vi "chart.vi"() -> ()   [LabVIEW 8.6]
uses:
  Controls/lxw_chart_type.ctl
  Controls/lxw_boolean.ctl
  Controls/lxw_defined_colors.ctl
panel:
  out "error out":errorcluster
  out "function return 2":string
  # "chart.xlsx"
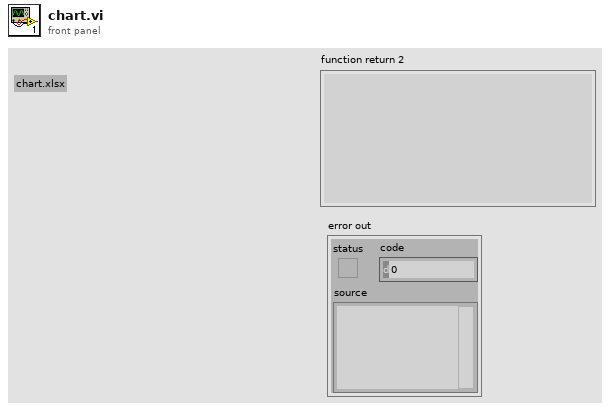
[diagram p1: front panel]
types:
  T1 = typedef "lxw_defined_colors.ctl" = u32
  T2 = typedef "lxw_boolean.ctl" = u8
  T3 = cluster{"name":u32, "@dummy control@":i8, "@dummy control@":i8, "@dummy control@":i8, "@dummy control@":i8, "size":dbl, "bold":u8, "italic":u8, "underline":u8, "@dummy control@":i8, "rotation":i32, "color":u32, "pitch_family":u8, "charset":u8, "baseline":i8}
  T4 = typedef "lxw_chart_type.ctl" = u8
  T5 = enum32{"invalid app kind", "Development System", "Run Time System", "Student Edition", "Embedded LabVIEW", "Evaluation", "Custom"}
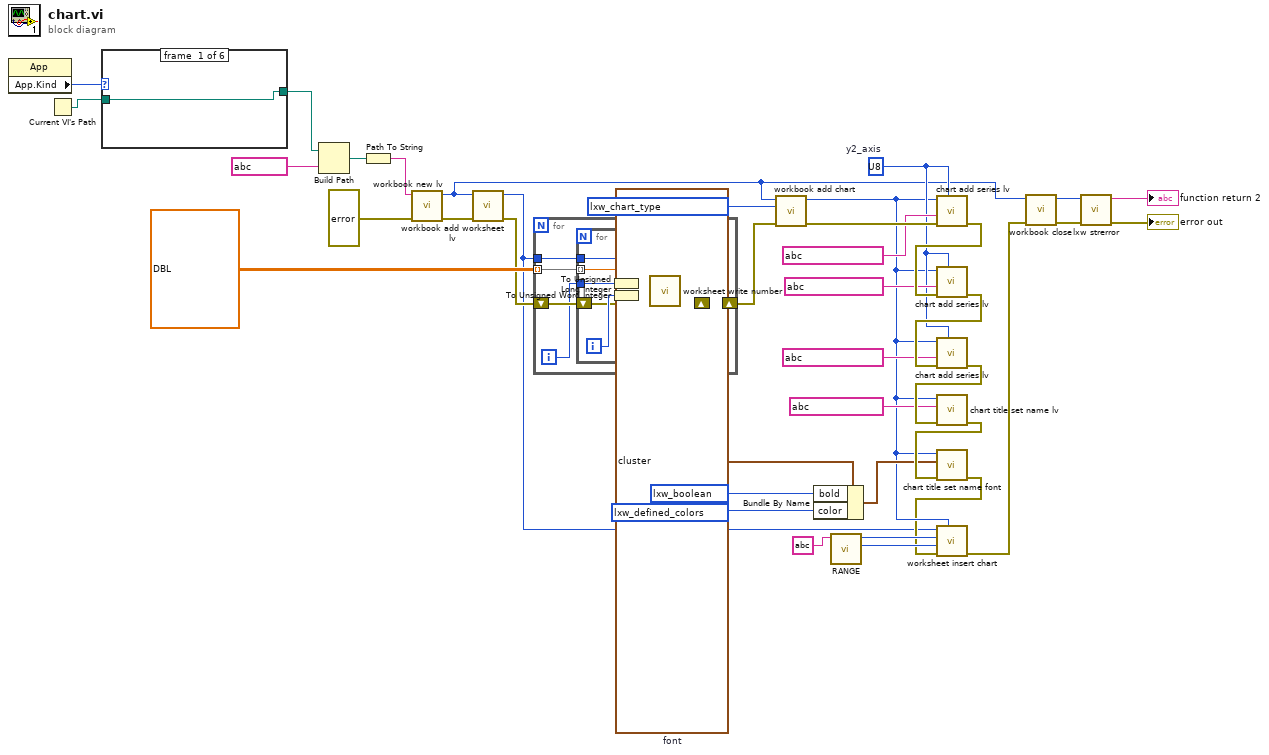
[diagram p0: block diagram]
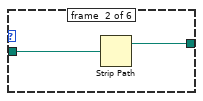
[diagram p2: hidden frame]
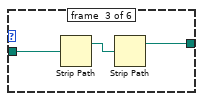
[diagram p3: hidden frame]
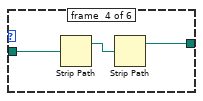
[diagram p4: hidden frame]
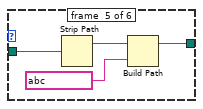
[diagram p5: hidden frame]
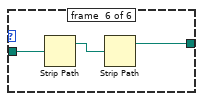
[diagram p6: hidden frame]
diagram:
  w9 = T1 ? items=["LXW_COLOR_BLACK", "LXW_COLOR_BLUE", "LXW_COLOR_BROWN", "LXW_COLOR_CYAN", "LXW_COLOR_GRAY", "LXW_COLOR_GREEN", "LXW_COLOR_LIME", "LXW_COLOR_MAGENTA", "LXW_COLOR_NAVY", "LXW_COLOR_ORANGE", "LXW_COLOR_PURPLE", "LXW_COLOR_RED", "LXW_COLOR_SILVER", "LXW_COLOR_WHITE", "LXW_COLOR_YELLOW"] ("Ring")
  w10 = T2 ? items=["LXW_FALSE", "LXW_TRUE", "LXW_EXPLICIT_FALSE"]
  w12 = T3 ?  # font
  w16 = u8 ?  # y2_axis
  w24 = T4 ? items=["LXW_CHART_NONE", "LXW_CHART_AREA", "LXW_CHART_AREA_STACKED", "LXW_CHART_AREA_STACKED_PERCENT", "LXW_CHART_BAR", "LXW_CHART_BAR_STACKED", "LXW_CHART_BAR_STACKED_PERCENT", "LXW_CHART_COLUMN", "LXW_CHART_COLUMN_STACKED", "LXW_CHART_COLUMN_STACKED_PERCENT", "LXW_CHART_DOUGHNUT", "LXW_CHART_LINE", "LXW_CHART_LINE_STACKED", "LXW_CHART_LINE_STACKED_PERCENT", "LXW_CHART_PIE", "LXW_CHART_SCATTER", "LXW_CHART_SCATTER_STRAIGHT", "LXW_CHART_SCATTER_STRAIGHT_WITH_MARKERS", "LXW_CHART_SCATTER_SMOOTH", "LXW_CHART_SCATTER_SMOOTH_WITH_MARKERS", "LXW_CHART_RADAR", "LXW_CHART_RADAR_WITH_MARKERS", "LXW_CHART_RADAR_FILLED", "LXW_CHART_STOCK"] ("chart_type")
  n1 = property class="App"() -> ("App.Kind"=w38:T5)  [unwired: 2 in, 2 out]
  n2 = Current VI's Path() -> (path=w37:path)
  n3 = case shown="\"Evaluation\"" w38 {
    tunnel: w37 -> [w39 w41 w44 w47 w51 w54]
    tunnel: [w39 w40 w42 w45 w49 w52] -> w36
    frame #0 {
    }
    frame #1 {
      n4 = Strip Path(path=w41) -> (stripped path=w40:path)  [unwired: 1 out]
    }
    frame #2 {
      n5 = Strip Path(path=w44) -> (stripped path=w43:path)  [unwired: 1 out]
      n6 = Strip Path(path=w43) -> (stripped path=w42:path)  [unwired: 1 out]
    }
    frame #3 {
      n7 = Strip Path(path=w47) -> (stripped path=w46:path)  [unwired: 1 out]
      n8 = Strip Path(path=w46) -> (stripped path=w45:path)  [unwired: 1 out]
    }
    frame #4 {
      n9 = Strip Path(path=w51) -> (stripped path=w50:path)  [unwired: 1 out]
      n10 = Build Path(base path=w50, name or relative path=string ?) -> (appended path=w49:path)
    }
    frame #5 {
      n11 = Strip Path(path=w54) -> (stripped path=w53:path)  [unwired: 1 out]
      n12 = Strip Path(path=w53) -> (stripped path=w52:path)  [unwired: 1 out]
    }
  }
  n13 = Build Path(base path=w36, name or relative path=string ? ("filename")) -> (appended path=w28:path)
  n14 = Path To String(path=w28) -> (string=w27:string)
  n15 = call "workbook new lv.vi"("error in (no error)"=errorcluster ?, "filename"=w27) -> ("error out"=w34:errorcluster, "function return"=w8:u32)  [unwired: 8 in]
  n16 = call "workbook add worksheet lv.vi"("error in (no error)"=w34, "workbook"=w8) -> ("error out"=w25:errorcluster, "function return"=w1:u32)  [unwired: 8 in]
  n17 = for {
    tunnel: dbl[][] ? -> [w59] mode=indexing
    shift-right: [w57] -> w22
    shift-left: w25 -> [w58]
    tunnel: w1 -> [w55]
    i -> [w56]
    n18 = for {
      tunnel: w59 -> [w67] mode=indexing
      tunnel: w56 -> [w64]
      shift-right: [w61] -> w57
      shift-left: w58 -> [w62]
      tunnel: w55 -> [w60]
      i -> [w66]
      n19 = To Unsigned Long Integer(number=w64) -> (unsigned 32bit integer=w63:u32)
      n20 = To Unsigned Word Integer(number=w66) -> (unsigned 16bit integer=w65:u16)
      n21 = call "worksheet write number.vi"("number"=w67, "error in (no error)"=w62, "col"=w65, "row"=w63, "worksheet"=w60) -> ("error out"=w61:errorcluster)  [unwired: 5 in, 1 out]
    }
  }
  n22 = call "workbook add chart.vi"("error in (no error)"=w22, "chart_type"=w24, "workbook"=w8) -> ("error out"=w23:errorcluster, "function return"=w7:u32)  [unwired: 7 in]
  n23 = Bundle By Name(cluster=w12, "bold"=w10, "color"=w9) -> (w11:T3)
  n24 = call "RANGE.vi"("range_str"=string ?) -> ("col"=w5:u16, "row"=w4:u32)  [unwired: 6 in, 3 out]
  n25 = call "chart add series lv.vi"("y2_axis"=w16, "error in (no error)"=w23, "values"=string ?, "chart"=w7) -> ("error out"=w21:errorcluster)  [unwired: 6 in, 1 out]
  n26 = call "chart add series lv.vi"("y2_axis"=w16, "error in (no error)"=w21, "values"=string ?, "chart"=w7) -> ("error out"=w20:errorcluster)  [unwired: 6 in, 1 out]
  n27 = call "chart add series lv.vi"("y2_axis"=w16, "error in (no error)"=w20, "values"=string ?, "chart"=w7) -> ("error out"=w15:errorcluster)  [unwired: 6 in, 1 out]
  n28 = call "chart title set name lv.vi"("error in (no error)"=w15, "name"=string ?, "chart"=w7) -> ("error out"=w13:errorcluster)  [unwired: 8 in]
  n29 = call "chart title set name font.vi"("error in (no error)"=w13, "font"=w11, "chart"=w7) -> ("error out"=w2:errorcluster)  [unwired: 7 in, 1 out]
  n30 = call "worksheet insert chart.vi"("chart"=w7, "error in (no error)"=w2, "col"=w5, "row"=w4, "worksheet"=w1) -> ("error out"=w6:errorcluster)  [unwired: 5 in, 1 out]
  n31 = call "workbook close.vi"("error in (no error)"=w6, "workbook"=w8) -> ("error out"=w30:errorcluster, "function return"=w32:u32)  [unwired: 8 in]
  n32 = call "lxw strerror.vi"("error in (no error)"=w30, "error_num"=w32) -> ("error out"=→"error out":errorcluster, "function return"=→"function return 2":string)  [unwired: 8 in]
